vi "MICS Response Lookup.vi"(0 "error in":errorcluster, 4 "Token":u8) -> (5 "row index":i32=-1, 6 "found":bool, 7 "error out":errorcluster, 8 "description":string, 9 "name":string)   [LabVIEW 2020]
doc: "This function searches the MICS Response Table indexed by Token, to find the corresponding Name and Description strings.\n\nThe MICS Repsonse Table is inported from SWEX 0091 Rev 1.8, SCS Error Codes and Command Responses, pages 19-23."
panel:
  in  "MICS Responses":string[][](table)=[["255", "0xFF", "COMMAND ACCEPTED", "The received command (identified in the response) was processed and performed without error. Any data to be returned as a result of the command completion is present in the response."], ["0", "0x00", "INVALID EXID", "The External ID contained in the command is for an external device the xPG has not been configured to process commands from."], ["1", "0x01", "INVALID COMMAND", "The Token in the received command is invalid/unknown to the xPG."], ["2", "0x02", "INVALID PARAM", "A parameter provided with the received command has been determined to be invalid and prohibits further processing of the command."], ["3", "0x03", "BUSY", "The xPG cannot execute the received command while in its present operational state.  Examples include: * Selecting program while stim on * Restoring program defaults while stim on * Writing to flash while stim on [CP commands] "], ["16", "0x10", "COMMAND NOT VALID WHILE IDLE", "The command is not valid when stimulation is not active.  (This code generally applies to commands that are used to modify stimulation.)"], ["17", "0x11", "COMMAND NOT VALID WHILE RAMPING", "The command is not valid when the xPG is ramping the stimulus amplitude immediately after turning stimulation on.  (This code generally applies to commands that are used to modify stimulation parameters)"], ["18", "0x12", "COMMAND LOCKED OUT (temporary)", "The command is temporarily locked out. (This code generally applies to commands that are used to modify stimulation, resulting in an increase in stimulation energy)"], ["19", "0x13", "DEPRECATED", ""], ["32", "0x20", "PROGRAM NOT VALID", "The command cannot be executed because the program definition is not valid.  A way to delete a program is to set it not valid.  Then when IPG returns valid programs bitmap it will not be listed as available."], ["33", "0x21", "PROGRAM DISABLED", "The command cannot be executed because the program definition has been disabled, due to a hardware issue."], ["34", "0x22", "BATTERY TOO LOW", "The xPG Stimulation command to turn stimulation on cannot be executed because the battery level is too low for safe stimulation.  IPG could have said battery was OK, but then dropped below threshold since having last sent status.  "], ["35", "0x23", "DEPRECATED –  Use 0x03 BUSY. ", ""], ["36", "0x24", "NO PROGRAM SELECTED", "The requested command (only in response to stim on) cannot be executed because no program is presently selected."], ["37", "0x25", "BOOST CONVERTER STARTUP FAILED", "Stimulation cannot be started because the high voltage boost converter did not initialize correctly."], ["38", "0x26", "PULSE GUARD CHECK FAILED", "Stimulation cannot be started because the pulse guard circuit check failed."], ["39", "0x27", "STIMULATION POWER ON FAILED", "Stimulation cannot be started because the stimulation chip failed to power up correctly."], ["40", "0x28", "ACTIVE RECOVERY DISABLED", "Stimulation cannot be started because automatic waveform adjustment failed."], ["41", "0x29", "DEPRECATED – Use 0x36 MOD VIOLATES ELECTRODE CHARGE DENSITY LIMIT", ""], ["42", "0x2A", "DEPRECATED – Use 0x02 INVALID PARAM.", ""], ["43", "0x2B", "DEPRECATED – USE 0x02 INVALID PARAM.", ""], ["44", "0x2C", "DEPRECATED – Use 0x02 INVALID PARAM.", ""], ["45", "0x2D", "DEPRECATED – Use 0x02 INVALID PARAM.", ""], ["46", "0x2E", "SETUP ERROR, BAD STIM ASIC READ-BACK", "While attempting to set-up the stim ASIC for output, the verification data read-back of certain registers did not match the set-up data. "], ["47", "0x2F", "SETUP ERROR, BAD POWER ASIC READ-BACK", "While attempting to configure the power ASIC, the verification data read-back of certain registers did not match the set-up data."], ["48", "0x30", "DEPRECATED – Not Used.", ""], ["49", "0x31", "ALL AMPLITUDES AT MINIMUM", "The Decrement Program Amplitude command cannot be executed because all pulse amplitudes are the minimum allowed setting."], ["50", "0x32", "ALL AMPLITUDES AT MAXIMUM", "The Increment Program Amplitude command cannot be executed because all pulse amplitudes are the maximum allowed setting."], ["51", "0x33", "PULSE NOT VALID", "The command to modify the specified pulse amplitude or pulse width cannot be executed because the pulse in not defined in the program that is running."], ["52", "0x34", "PULSE WIDTH EXCEEDS LIMITS", "The requested pulse width modification command cannot be executed because it would exceed the programmed pulse width limits for the specified pulse."], ["53", "0x35", "DEPRECATED - Use 0x02 INVALID PARAM.", ""], ["54", "0x36", "MOD VIOLATES ELECTRODE CHARGE DENSITY LIMIT", "The requested pulse output modification cannot be executed because it would violate the charge density limit for one or more of the selected electrode channels."], ["55", "0x37", "MOD VIOLATES ELECTRODE CURRENT DENSITY LIMIT", "The requested pulse output modification cannot be executed because it would violate the current density limit for one or more of the selected electrode channels."], ["56", "0x38", "PULSE WIDTH FREQUENCY CONFLICT", "* The requested pulse width increase cannot be executed because the program cannot be implemented at the specified program frequency. * The requested program frequency increase cannot be executed because the program cannot be implemented with the specified pulse widths. * The requested Test Pulse will not fit in the selected program period. * The requested pulse output requires active recovery, but the KrecsEnabledBitMap in the Pulse Constants is 0 (no krecs enabled). * The requested pulse output requires active recovery, but there are no krecs enabled (KrecsEnabledBitMap in Pulse Constants) that will fit the selected program period. "], ["57", "0x39", "DEPRECATED – Use PULSE WIDTH FREQUENCY CONFLICT", ""], ["58", "0x3A", "FREQUENCY MOD NOT ALLOWED", "The requested program frequency change is not allowed per the program definition.  (This could be because the specified frequency is not allowed or there is no frequency index lower or higher than the present index allowed.)"], ["59", "0x3B", "PULSE AMPLITUDE EXCEEDS LIMITS", "The requested pulse amplitude change cannot be executed because it would exceed the allowed limits for the specified pulse."], ["60", "0x3C", "DEPRECATED – Command n long exists", ""], ["64", "0x40", "TIMED OUT", "The operation requested timed out waiting for hardware to respond.  This response includes when an ADC read fails or when background impedance check fails to respond with a value."], ["85", "0x55", "CHARGING CONTROL ERROR", "An error occurred reading the temperature or battery level."], ["96", "0x60", "DATA CORRUPTED", "The requested Get Data command failed, or the requested data was detected as corrupt."], ["97", "0x61", "PROGRAM DEFINITION CORRUPTED", "The data integrity check for the program definition data for the requested program failed. IPG should set active error to PROGRAM DEFINITION CORRUPTED"], ["98", "0x62", "PROGRAM ACTIVE SETTINGS CORRUPTED", "The data integrity check for the active settings for the requested program failed.  IPG should set active error to PROGRAM ACTIVE SETTINGS CORRUPTED.  IPG will also return that active settings to default settings."], ["99", "0x63", "PROGRAM CONSTANTS CORRUPTED", "The data integrity check for the Program Constants data failed.  xPG should set active error to CRITICAL NV DATA CORRUPTED."], ["100", "0x64", "PULSE CONSTANTS CORRUPTED", "The data integrity check for the Pulse Constants data failed.  xPG should set active error to CRITICAL NV DATA CORRUPTED."], ["101", "0x65", "CHANNEL CALIBRATIONS CORRUPTED", "The data integrity check for the Channel Calibrations data failed.  xPG should set active error to CRITICAL NV DATA CORRUPTED."], ["102", "0x66", "LEAD LIMITS CORRUPTED", "The data integrity check for the Lead Limits data failed.  xPG should set active error to CRITICAL NV DATA CORRUPTED."], ["103", "0x67", "STIM ASIC HV CALIBRATIONS CORRUPTED", "The data integrity check for the Stim Asic HV Calibrations data failed.  xPG should set active error to CRITICAL NV DATA CORRUPTED."], ["104", "0x68", "RAMP TIME CORRUPTED", "The data integrity check for the Ramp Time failed.  xPG should set active error to CRITICAL NV DATA CORRUPTED."], ["105", "0x69", "DEPRECATED", ""], ["106", "0x6A", "DEPRECATED – Not Used", ""], ["112", "0x70", "FEATURE NOT ENABLED", "The requested feature is not presently enabled."], ["113", "0x71", "DEPRECATED - Use 0x02 INVALID PARAM.", ""], ["114", "0x72", "DEPRECATED - Use 0x02 INVALID PARAM.", ""], ["115", "0x73", "DEPRECATED – Use 0x03 BUSY.", ""], ["116", "0x74", "DEPRECATED – Use 0x38 PULSE WIDTH FREQUENCY CONFLICT", ""], ["117", "0x75", "DEPRECATED – Use 0x38 PULSE WIDTH FREQUENCY CONFLICT", ""], ["118", "0x76", "DEPRECATED – Use 0x38 PULSE WIDTH FREQUENCY CONFLICT", ""], ["119", "0x77", "WRITE FAILED", "The command failed while attempting to write data to memory or registers. Writes to flash shall use more specific error codes from the range below."], ["120", "0x78", "READ FAILED", "The command failed while attempting to read data to memory or registers. Reads to flash shall use more specific error codes from the range below."], ["121", "0x79", "DEPRECATED – Not Used", ""], ["128", "0x80", "DEPRECATED – Not Used", ""], ["129", "0x81", "BACKGROUND IMPEDANCE CHECK FAILED", "Pre-stimulation background impedance checks have failed.  This shall result in a Category 2 Error being reported."], ["130", "0x82", "BASIC OUTPUT CHECK FAILED", "Pre-stimulation basic output checks have failed.  This shall result in a Category 2 Error being reported."], ["131", "0x83", "STIM FAILED UNKNOWN SOFTWARE ERROR", "Stimulation has failed because of a software logic error.  Stimulation cannot be started."], ["132", "0x84", "STIMULATION FAILED – SEVERE ERROR EXISTS", "Stimulation has failed because a Category 1 error exists.  Stimulation cannot be started if such an error exists."], ["133", "0x85", "DEPRECATED – Not Used", ""], ["176", "0xB0", "FLASH ERROR INVALID ADDRESS", "Illegal flash address segment write.  The requested programming command failed while attempting to save data to the xPG’s non-volatile memory."], ["177", "0xB1", "FLASH ERROR SEGMENT BOUNDARY", "Requested flash address write overlaps segment boundary.  The requested programming command failed while attempting to save data to the xPG’s non-volatile memory."], ["178", "0xB2", "DEPRECATED – Use 0xB0 FLASH ERROR INVALID ADDRESS", "Invalid flash address reported while preparing for erasing segment.  The requested programming command failed while attempting to save data to the xPG’s non-volatile memory."], ["179", "0xB3", "FLASH ERASE ERROR FLASH CONTROLLER BUSY", "Flash controller unexpectedly reported busy while preparing for segment erase.  The requested programming command failed while attempting to save data to the xPG’s non-volatile memory."], ["180", "0xB4", "FLASH ERASE ERROR FLASH CONTROLLER SETUP", "Firmware setup error reported while preparing for segment erase.  The requested programming command failed while attempting to save data to the xPG’s non-volatile memory."], ["181", "0xB5", "FLASH ERASE ERROR TIMEOUT", "Busy bit timeout reported while waiting for segment erase. The requested programming command failed while attempting to save data to the xPG’s non-volatile memory."], ["182", "0xB6", "FLASH ERASE ERROR FAIL FLAG", "Fail flag set during segment erase.  The requested programming command failed while attempting to save data to the xPG’s non-volatile memory."], ["183", "0xB7", "FLASH ERASE ERROR ACCESS VIOLATION FLAG", "Access violation reported while attempting to erase flash.  The requested programming command failed while attempting to save data to the xPG’s non-volatile memory."], ["184", "0xB8", "FLASH ERASE ERROR BAD ERASE", "Segment not erased and segment erase reported as completed.  The requested programming command failed while attempting to save data to the xPG’s non-volatile memory."], ["192", "0xC0", "DEPRECATED – Use 0xB0 FLASH ERROR INVALID ADDRESS", ""], ["193", "0xC1", "FLASH WRITE ERROR FLASH CONTROLLER BUSY", "The flash controller reports unexpectedly busy while preparing for block write.  The requested programming command failed while attempting to save data to the xPG’s non-volatile memory."], ["194", "0xC2", "FLASH WRITE ERROR FLASH CONTROLLER SETUP", "A firmware setup error occurred while preparing for block write.  The requested programming command failed while attempting to save data to the xPG’s non-volatile memory."], ["195", "0xC3", "FLASH WORD WRITE ERROR TIMEOUT", "Wait bit timeout occurred while writing word to flash memory.  The requested programming command failed while attempting to save data to the xPG’s non-volatile memory."], ["196", "0xC4", "FLASH  WORD WRITE ERROR FAIL FLAG", "Flash fail flag set while writing word to flash memory.  The requested programming command failed while attempting to save data to the xPG’s non-volatile memory."], ["197", "0xC5", "FLASH WORD WRITE ERROR ACCESS VIOLATION", "Access violation reported while writing word to flash memory.  The requested programming command failed while attempting to save data to the xPG’s non-volatile memory."], ["198", "0xC6", "FLASH BLOCK WRITE ERROR TIMEOUT", "Wait bit timeout occurred while writing block to flash memory.  The requested programming command failed while attempting to save data to the xPG’s non-volatile memory."], ["199", "0xC7", "FLASH  BLOCK WRITE ERROR FAIL FLAG", "Flash fail flag set while writing block to flash memory.  The requested programming command failed while attempting to save data to the xPG’s non-volatile memory."], ["200", "0xC8", "FLASH BLOCK WRITE ERROR ACCESS VIOLATION", "Access violation reported while writing block to flash memory.  The requested programming command failed while attempting to save data to the xPG’s non-volatile memory."], ["201", "0xC9", "FLASH WRITE ERROR BAD WRITE", "After segment write completed, the flash destination data did not match the source data.  The requested programming command failed while attempting to save data to the xPG’s non-volatile memory."], ["202", "0xCA", "RESERVED – Not Used.", ""], ["203", "0xCB", "RESERVED – Not Used.", ""], ["204", "0xCC", "RESERVED – Not Used.", ""], ["205", "0xCD", "RESERVED – Not Used.", ""], ["206", "0xCE", "RESERVED – Not Used.", ""], ["207", "0xCF", "RESERVED – Not Used.", ""], ["-1", "Default", "ANY ERROR NOT LISTED HEREIN", "Undefined and unexpected.   "]]
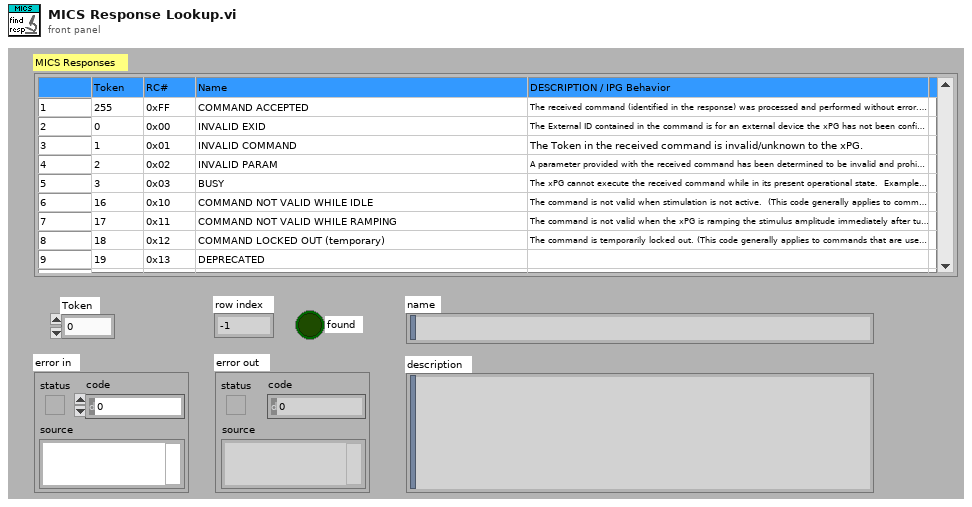
[diagram p1: front panel]
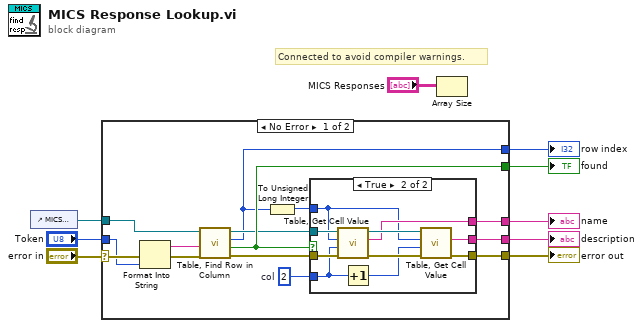
[diagram p0: block diagram]
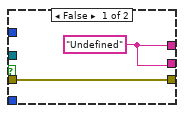
[diagram p2: hidden frame]
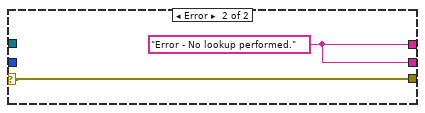
[diagram p3: hidden frame]
diagram:
  # "Connected to avoid compiler warnings."
  n1 = control-ref of="MICS Responses"() -> (w1:refnum<vi>)
  n2 = case shown="No Error" "error in" {
    selector: "error in" -> [w13 w37]
    tunnel: w1 -> [w23 _]
    tunnel: "Token" -> [w11 _]
    tunnel: [w21 w37] -> w8
    tunnel: [w20 _] -> w7
    tunnel: [w18 w36] -> w6
    tunnel: [w17 w36] -> w5
    tunnel: [w16 _] -> w4
    frame No Error {
      w14 = u32 2  # col
      n3 = Format Into String(error in=w13, w11) -> (resulting string=w10:string, error out=w12:errorcluster)  [unwired: 2 in]
      n4 = call "Table, Find Row in Column.vi"("error in"=w12, "search key"=w10, "Tbl Refnum"=w23) -> ("error out"=w22:errorcluster, "found"=w20:bool, "row index"=w16:i32, "Tbl Refnum out"=w19:refnum<vi>)  [unwired: 5 in]
      n5 = To Unsigned Long Integer(number=w16) -> (unsigned 32bit integer=w15:u32)
      n6 = case shown="True" w20 {
        tunnel: w22 -> [w25 w35]
        tunnel: [w25 w33] -> w21
        tunnel: w19 -> [_ w32]
        tunnel: [w24 w30] -> w18
        tunnel: [w24 w29] -> w17
        tunnel: w15 -> [_ w27]
        tunnel: w14 -> [_ w26]
        frame False {
          w24 = "Undefined" ("cell value")
        }
        frame True {
          n7 = call "Table, Get Cell Value.vi"("error in"=w35, "column (0)"=w26, "row (0)"=w27, "Tbl Refnum"=w32) -> ("error out"=w34:errorcluster, "cell value"=w29:string, "Tbl Refnum out"=w31:refnum<vi>)  [unwired: 5 in]
          n8 = Increment(x=w26) -> (x+1=w28:u32)
          n9 = call "Table, Get Cell Value.vi"("error in"=w34, "column (0)"=w28, "row (0)"=w27, "Tbl Refnum"=w31) -> ("error out"=w33:errorcluster, "cell value"=w30:string)  [unwired: 5 in, 1 out]
        }
      }
    }
    frame Error {
      w36 = "Error - No lookup performed." ("cell value")
    }
  }
  "error out" <- w8
  "row index" <- w4
  "found" <- w7
  "name" <- w5
  "description" <- w6
  n10 = Array Size(array="MICS Responses") -> ()  [unwired: 1 out]
